vi "Run Bfr Rx - PingPongSized - Change Buffer.vi"(7 "Buffer_A":u64 format="%016x", 8 "error in (no error)":errorcluster, 11 "Ping Pong Buffer in":T1 {"Active Buffer Ref" format="%016x"}) -> (0 "error out":errorcluster, 3 "Ping Pong Buffer out":T1 {"Active Buffer Ref" format="%016x"})   [LabVIEW 2016, in "UDP-Custom-Device Engine.lvlib"]
uses:
  UDP-Custom-Device Engine.lvlib
  Types/Engine - Buffered Rx Ping Pong Buffer.ctl
  Types/Engine - Buffered Rx Active Buffer.ctl
  <vilib>/NI Veristand/VeriStand Data/Pointer Operations/Pointer.Write (U8).vi
  <vilib>/NI Veristand/VeriStand Data/VeriStand Data.lvlib
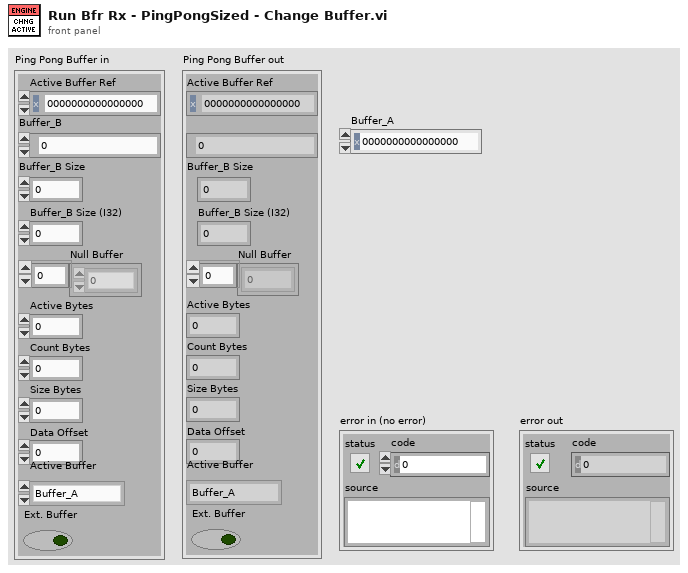
[diagram p1: front panel]
types:
  T1 = typedef "UDP-Custom-Device Engine.lvlib/Engine - Buffered Rx Ping Pong Buffer.ctl" = cluster{"Active Buffer Ref":u64, "Buffer_B":u64, "Buffer_B Size":u64, "Buffer_B Size (I32)":i32, "Null Buffer":u8[], "Active Bytes":u64, "Count Bytes":u64, "Size Bytes":u64, "Data Offset":u64, "Active Buffer":T2, "Ext. Buffer":bool}
  T2 = typedef "UDP-Custom-Device Engine.lvlib/Engine - Buffered Rx Active Buffer.ctl" = enum16{"Buffer_A", "Buffer_B"}
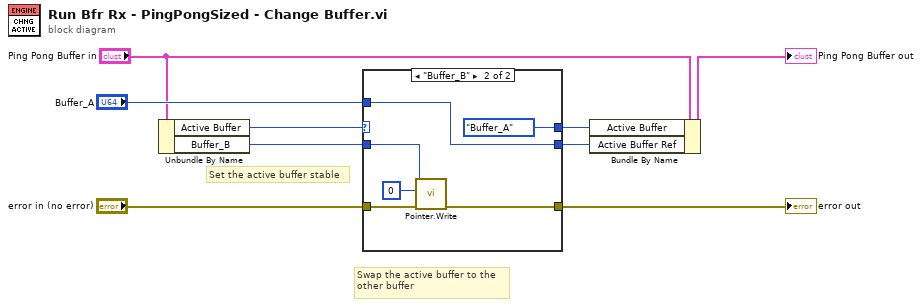
[diagram p0: block diagram]
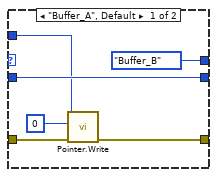
[diagram p2: hidden frame]
diagram:
  # "Swap the active buffer to the\nother buffer"
  # "Set the active buffer stable"
  n1 = Unbundle By Name("Ping Pong Buffer in") -> ("Active Buffer"=w9:T2, "Buffer_B"=w8:u64)
  n2 = case shown="\"Buffer_B\"" w9 {
    tunnel: w8 -> [w15 w16]
    tunnel: "Buffer_A" -> [w10 w21]
    tunnel: [w11 w17] -> w6
    tunnel: "error in (no error)" -> [w12 w18]
    tunnel: [w15 w21] -> w5
    tunnel: [Engine_-_Buffered_Rx_Active_Buffer."Buffer_B" ("Active Buffer") Engine_-_Buffered_Rx_Active_Buffer."Buffer_A" ("Active Buffer")] -> w2
    frame "Buffer_A", Default {
      n3 = call-poly <vilib>:"Pointer.Write.vi"("error in (no error)"=w12, "value"=u8 0, "pointer in"=w10) -> ("error out"=w11:errorcluster)  [unwired: 6 in, 2 out]
    }
    frame "Buffer_B" {
      n4 = call-poly <vilib>:"Pointer.Write.vi"("error in (no error)"=w18, "value"=u8 0, "pointer in"=w16) -> ("error out"=w17:errorcluster)  [unwired: 6 in, 2 out]
    }
  }
  "error out" <- w6
  n5 = Bundle By Name(cluster="Ping Pong Buffer in", "Active Buffer"=w2, "Active Buffer Ref"=w5) -> (→"Ping Pong Buffer out":T1)
